vi "Write AllowRTPopup.vi"(5 "AllowRTPopup":bool, 9 "FPWindow in":refnum<class "FPWindow.lvclass">) -> (3 "FPWindow out":refnum<class "FPWindow.lvclass">)   [LabVIEW 2014, in "FPWindow.lvclass"]
uses:
  FPWindow.lvclass
  FPWindow.lvclass/FPWindow.ctl
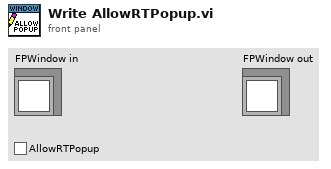
[diagram p1: front panel]
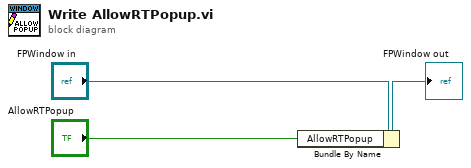
[diagram p0: block diagram]
diagram:
  n1 = Bundle By Name(cluster="FPWindow in", "AllowRTPopup"="AllowRTPopup") -> (→"FPWindow out":refnum<class "FPWindow.lvclass">)
